vi "Write kickTarget.vi"(8 "error in (no error)":errorcluster, 10 "kickTarget":dbl[](array[numeric]), 11 "PrimaryAttackerRole in":refnum<class "PrimaryAttackerRole.lvclass">) -> (0 "error out":errorcluster, 3 "PrimaryAttackerRole out":refnum<class "PrimaryAttackerRole.lvclass">)   [LabVIEW 2023, in "PrimaryAttackerRole.lvclass"]
uses:
  PrimaryAttackerRole.lvclass
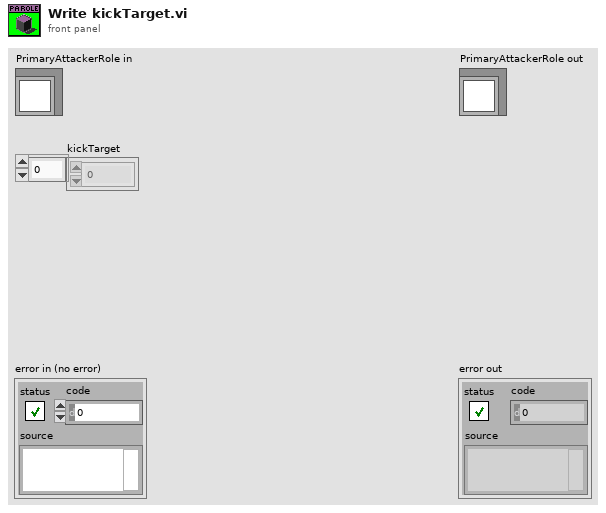
[diagram p1: front panel]
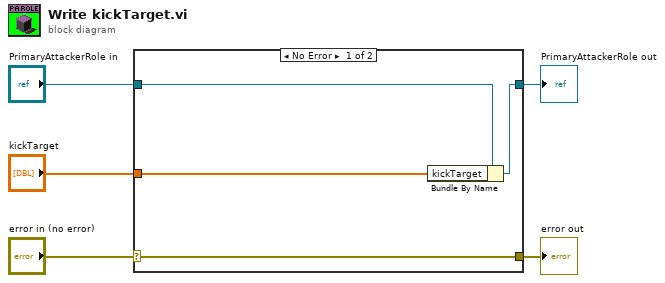
[diagram p0: block diagram]
diagram:
  n1 = case shown="No Error" "error in (no error)" {
    selector: "error in (no error)" -> [w9 w10]
    tunnel: [w9 w10] -> w4
    tunnel: [w7 w11] -> w2
    tunnel: "PrimaryAttackerRole in" -> [w8 w11]
    tunnel: "kickTarget" -> [w6 _]
    frame No Error {
      n2 = Bundle By Name(cluster=w8, "kickTarget"=w6) -> (w7:refnum<class "PrimaryAttackerRole.lvclass">)
    }
    frame Error {
    }
  }
  "error out" <- w4
  "PrimaryAttackerRole out" <- w2
